vi "ErrorCalulation.vi"(10 "desired x y theta":cluster{"xd":dbl, "yd":dbl, "thetad":dbl}, 11 "real x y theta":cluster{"xr":dbl, "yr":dbl, "thetar":dbl}) -> (9 "error":cluster{"xe":dbl, "ye":dbl, "thetae":dbl})   [LabVIEW 2016]
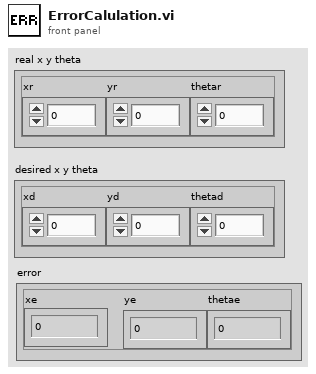
[diagram p1: front panel]
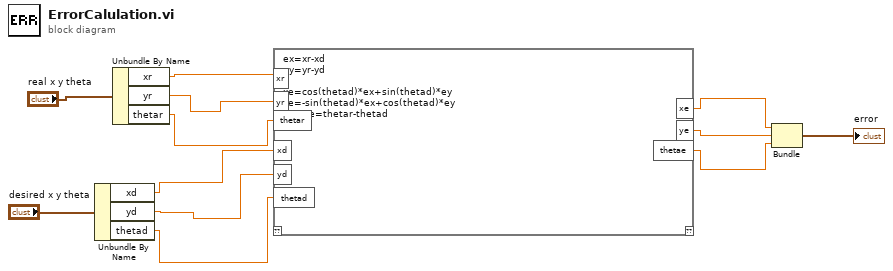
[diagram p0: block diagram]
diagram:
  n1 = Unbundle By Name("desired x y theta") -> ("xd"=w7:dbl, "yd"=w6:dbl, "thetad"=w5:dbl)
  n2 = Unbundle By Name("real x y theta") -> ("xr"=w11:dbl, "yr"=w10:dbl, "thetar"=w9:dbl)
  n3 = script code="ex=xr-xd\ney=yr-yd\n\nxe=cos(thetad)*ex+sin(thetad)*ey\nye=-sin(thetad)*ex+cos(thetad)*ey\nthetae=thetar-thetad"("xr"=w11, "yr"=w10, "thetar"=w9, "xd"=w7, "yd"=w6, "thetad"=w5) -> ("xe"=w4:dbl, "ye"=w3:dbl, "thetae"=w2:dbl)  [unwired: 1 in, 1 out]
  n4 = Bundle(w4, w3, w2) -> (→"error":cluster{dbl, dbl, dbl})  [unwired: 1 in]
